vi "Brick Dispenser.vi"() -> ()   [LabVIEW 2012]
panel:
  in  "?":bool
  in  "?":bool
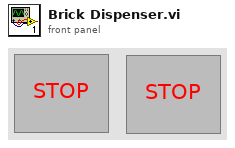
[diagram p1: front panel]
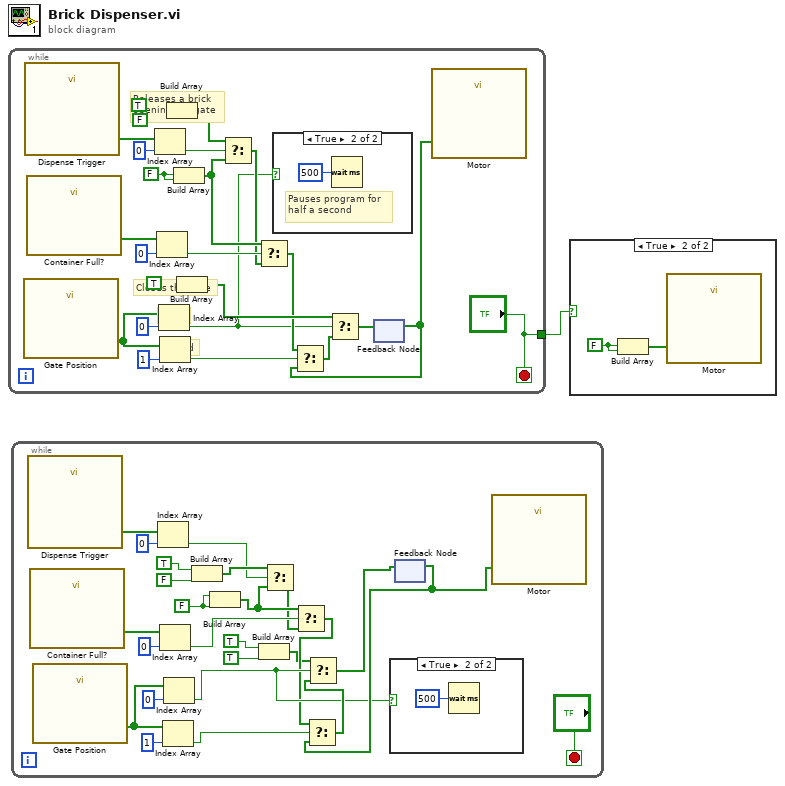
[diagram p0: block diagram]
diagram:
  n1 = while {
    tunnel: ["?"] -> w1
    stop <- "?" stop-if-true
    w10 = TRUE
    w12 = FALSE
    # "Closes the gate"
    # "Releases a brick\nopening the gate"
    # "Closed"
    # "Open"
    n2 = call "Gate Position"() -> ("data"=w20:bool[])  [unwired: 17 in, 2 out]
    n3 = call "Dispense Trigger"() -> ("data"=w25:bool[])  [unwired: 17 in, 2 out]
    n4 = call "Container Full?"() -> ("data"=w22:bool[])  [unwired: 17 in, 2 out]
    n5 = Index Array(array=w25, index=0) -> (element=w17:bool)
    n6 = Index Array(array=w22, index=0) -> (element=w16:bool)
    n7 = Index Array(array=w20, index=0) -> (element=w3:bool)
    n8 = Index Array(array=w20, index=1) -> (element=w18:bool)
    n9 = Build Array(TRUE, FALSE) -> (w13:bool[])
    n10 = Build Array(w12, w12) -> (w11:bool[])
    n11 = Build Array(w10, w10) -> (w9:bool[])
    n12 = Select(t=w13, s=w17, f=w11) -> (s? t:f=w7:bool[])
    n13 = Select(t=w11, s=w16, f=w7) -> (s? t:f=w8:bool[])
    n14 = case shown="True" w3 {
      frame False {
      }
      frame True {
        # "Pauses program for\nhalf a second"
        n15 = Wait (ms)(milliseconds to wait=u32 500) -> ()  [unwired: 1 out]
      }
    }
    n16 = feedback #1() -> (w4:bool[])  [unwired: 1 in]
    n17 = Select(t=w8, s=w18, f=w4) -> (s? t:f=w6:bool[])
    n18 = Select(t=w9, s=w3, f=w6) -> (s? t:f=w5:bool[])
    n19 = feedback-in #1(w5) -> ()
    n20 = call "Motor"("data"=w4) -> ()  [unwired: 17 in, 2 out]
  }
  n21 = while {
    stop <- "?" stop-if-true
    w39 = FALSE
    n22 = call "Dispense Trigger"() -> ("data"=w27:bool[])  [unwired: 17 in, 2 out]
    n23 = call "Container Full?"() -> ("data"=w48:bool[])  [unwired: 17 in, 2 out]
    n24 = call "Gate Position"() -> ("data"=w45:bool[])  [unwired: 17 in, 2 out]
    n25 = Index Array(array=w27, index=0) -> (element=w31:bool)
    n26 = Index Array(array=w48, index=0) -> (element=w37:bool)
    n27 = Index Array(array=w45, index=1) -> (element=w44:bool)
    n28 = Index Array(array=w45, index=0) -> (element=w38:bool)
    n29 = Build Array(TRUE, FALSE) -> (w35:bool[])
    n30 = Build Array(w39, w39) -> (w34:bool[])
    n31 = Build Array(TRUE, TRUE) -> (w28:bool[])
    n32 = Select(t=w35, s=w31, f=w34) -> (s? t:f=w33:bool[])
    n33 = Select(t=w34, s=w37, f=w33) -> (s? t:f=w36:bool[])
    n34 = case shown="True" w38 {
      frame False {
      }
      frame True {
        n35 = Wait (ms)(milliseconds to wait=u32 500) -> ()  [unwired: 1 out]
      }
    }
    n36 = feedback #2() -> (w40:bool[])  [unwired: 1 in]
    n37 = Select(t=w36, s=w44, f=w40) -> (s? t:f=w41:bool[])
    n38 = Select(t=w28, s=w38, f=w41) -> (s? t:f=w32:bool[])
    n39 = feedback-in #2(w32) -> ()
    n40 = call "Motor"("data"=w40) -> ()  [unwired: 17 in, 2 out]
  }
  n41 = case shown="True" w1 {
    frame False {
    }
    frame True {
      w54 = FALSE
      n42 = Build Array(w54, w54) -> (w53:bool[])
      n43 = call "Motor"("data"=w53) -> ()  [unwired: 17 in, 2 out]
    }
  }
